vi "Relative Path to Absolute Path.vi"(5 "Relative Path":path) -> (2 "Absolute Path":path)   [LabVIEW 2020, in "RxnRover.lvlib" / "File IO.lvlib"]
uses:
  File IO.lvlib
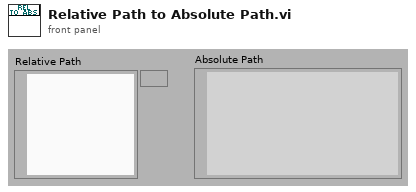
[diagram p1: front panel]
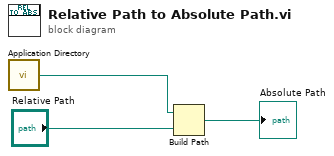
[diagram p0: block diagram]
diagram:
  n1 = call <vilib>:"Application Directory.vi"() -> ("Application Directory"=w1:path)
  n2 = Build Path(base path=w1, name or relative path="Relative Path") -> (appended path=→"Absolute Path":path)
